vi "washingermmachine.vi"() -> ()   [LabVIEW 2024]
panel:
  out "String 2":string
  out "bytes to read 6":i32
  in  "stop 6":bool
  out "Timer 2":dbl
  out "Water Temp 2":dbl(slide) scale=20.0..60.0
  out "bytes to read 5":i32
  in  "stop 5":bool
  out "Water Level 2":dbl(slide) scale=20.0..60.0
  out "bytes to read 4":i32
  in  "stop 4":bool
  out "Boolean 2":bool
  out "String":string
  out "Timer":dbl
  out "bytes to read 3":i32
  in  "stop 3":bool
  out "Water Temp":dbl(slide) scale=20.0..60.0
  out "bytes to read 2":i32
  in  "stop 2":bool
  in  "stop":bool
  out "bytes to read":i32
  out "Water Level":dbl(slide) scale=20.0..60.0
  out "Boolean":bool
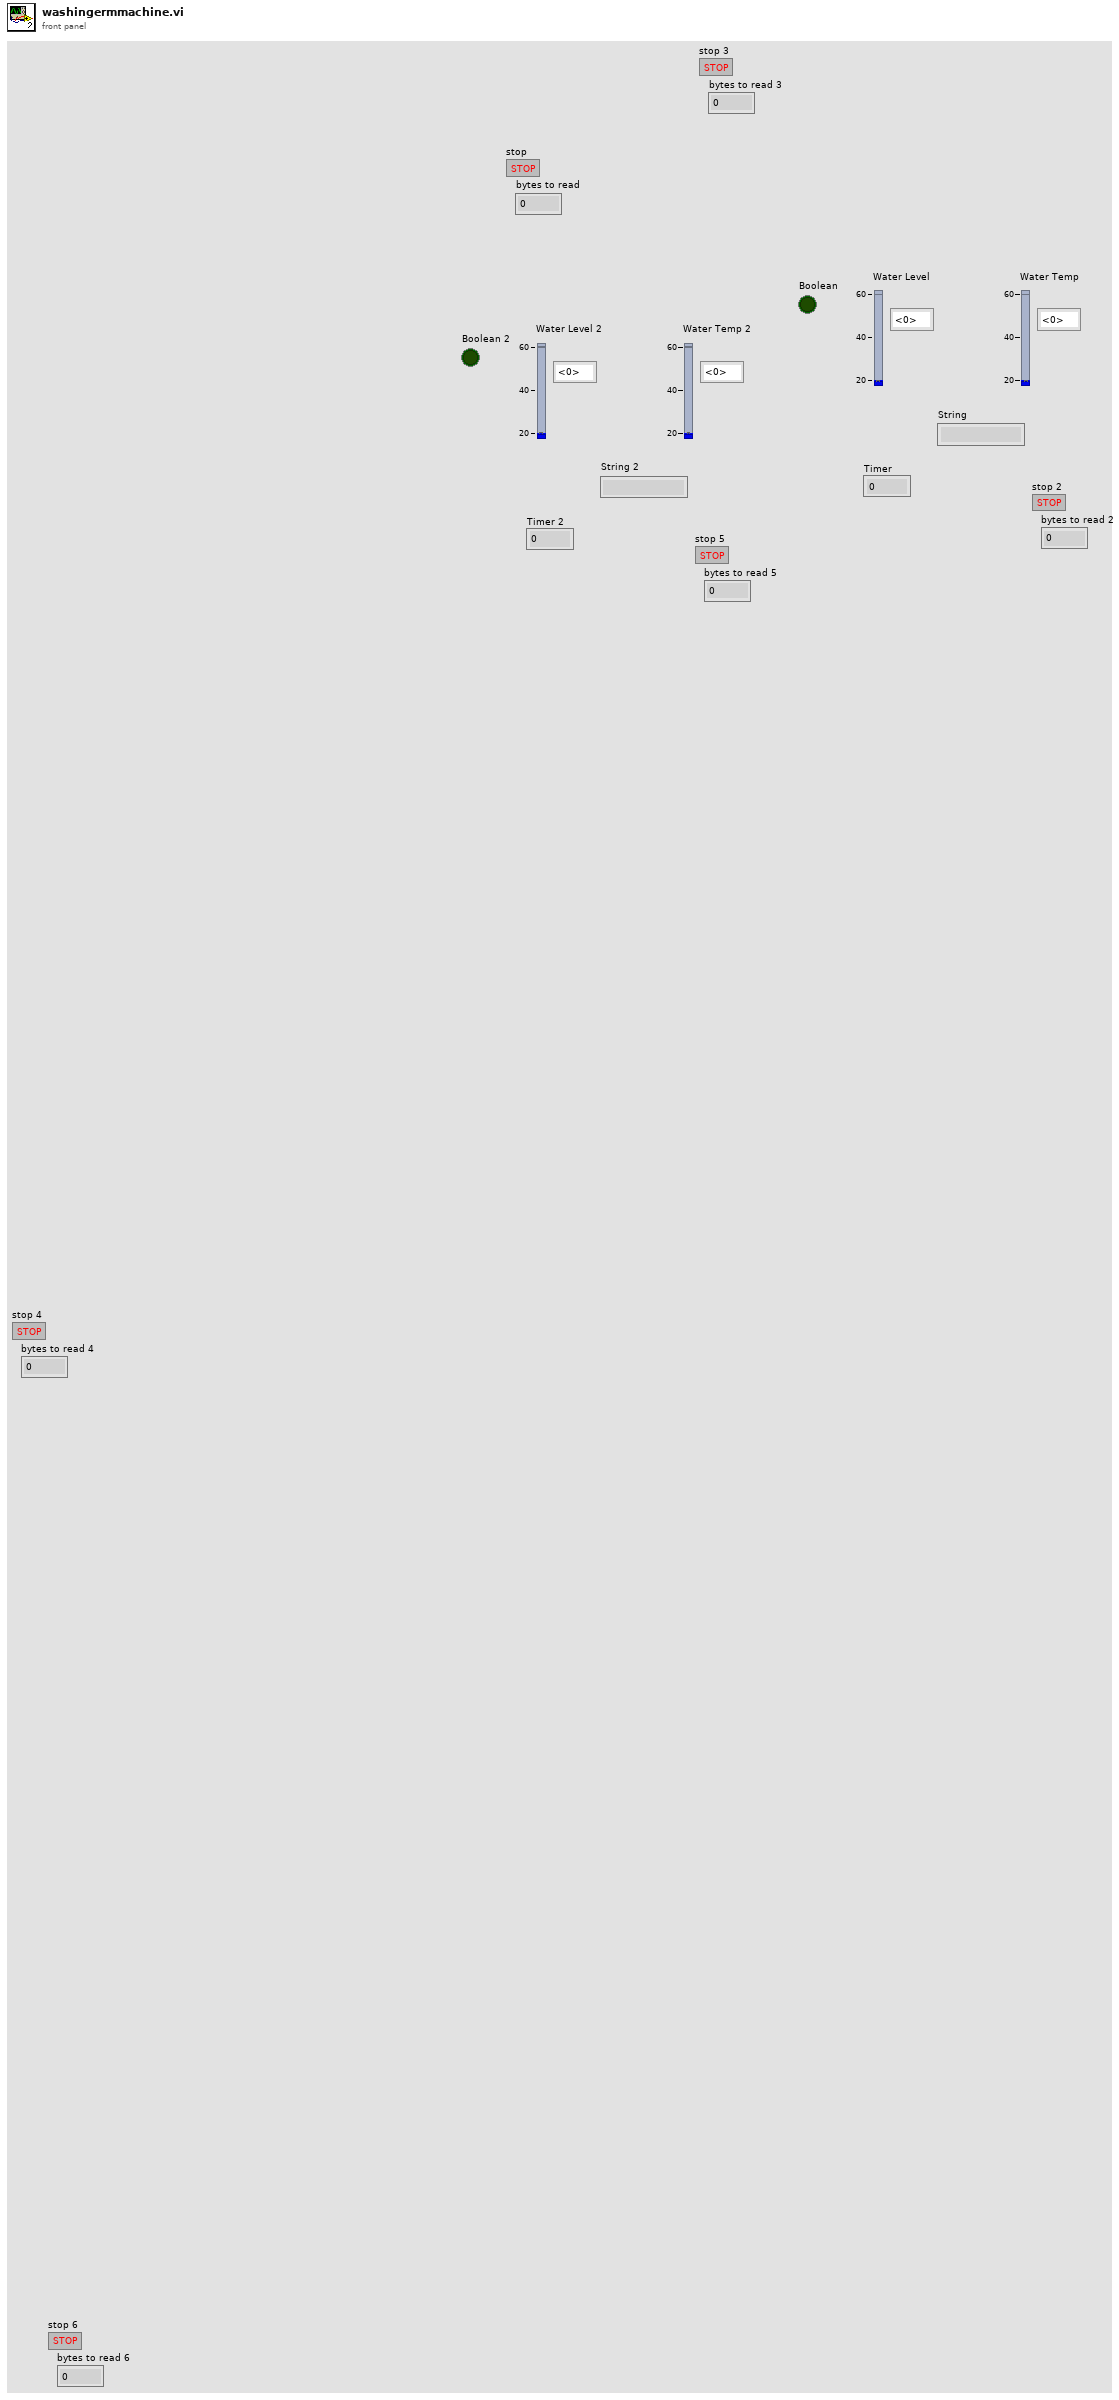
[diagram p1: front panel]
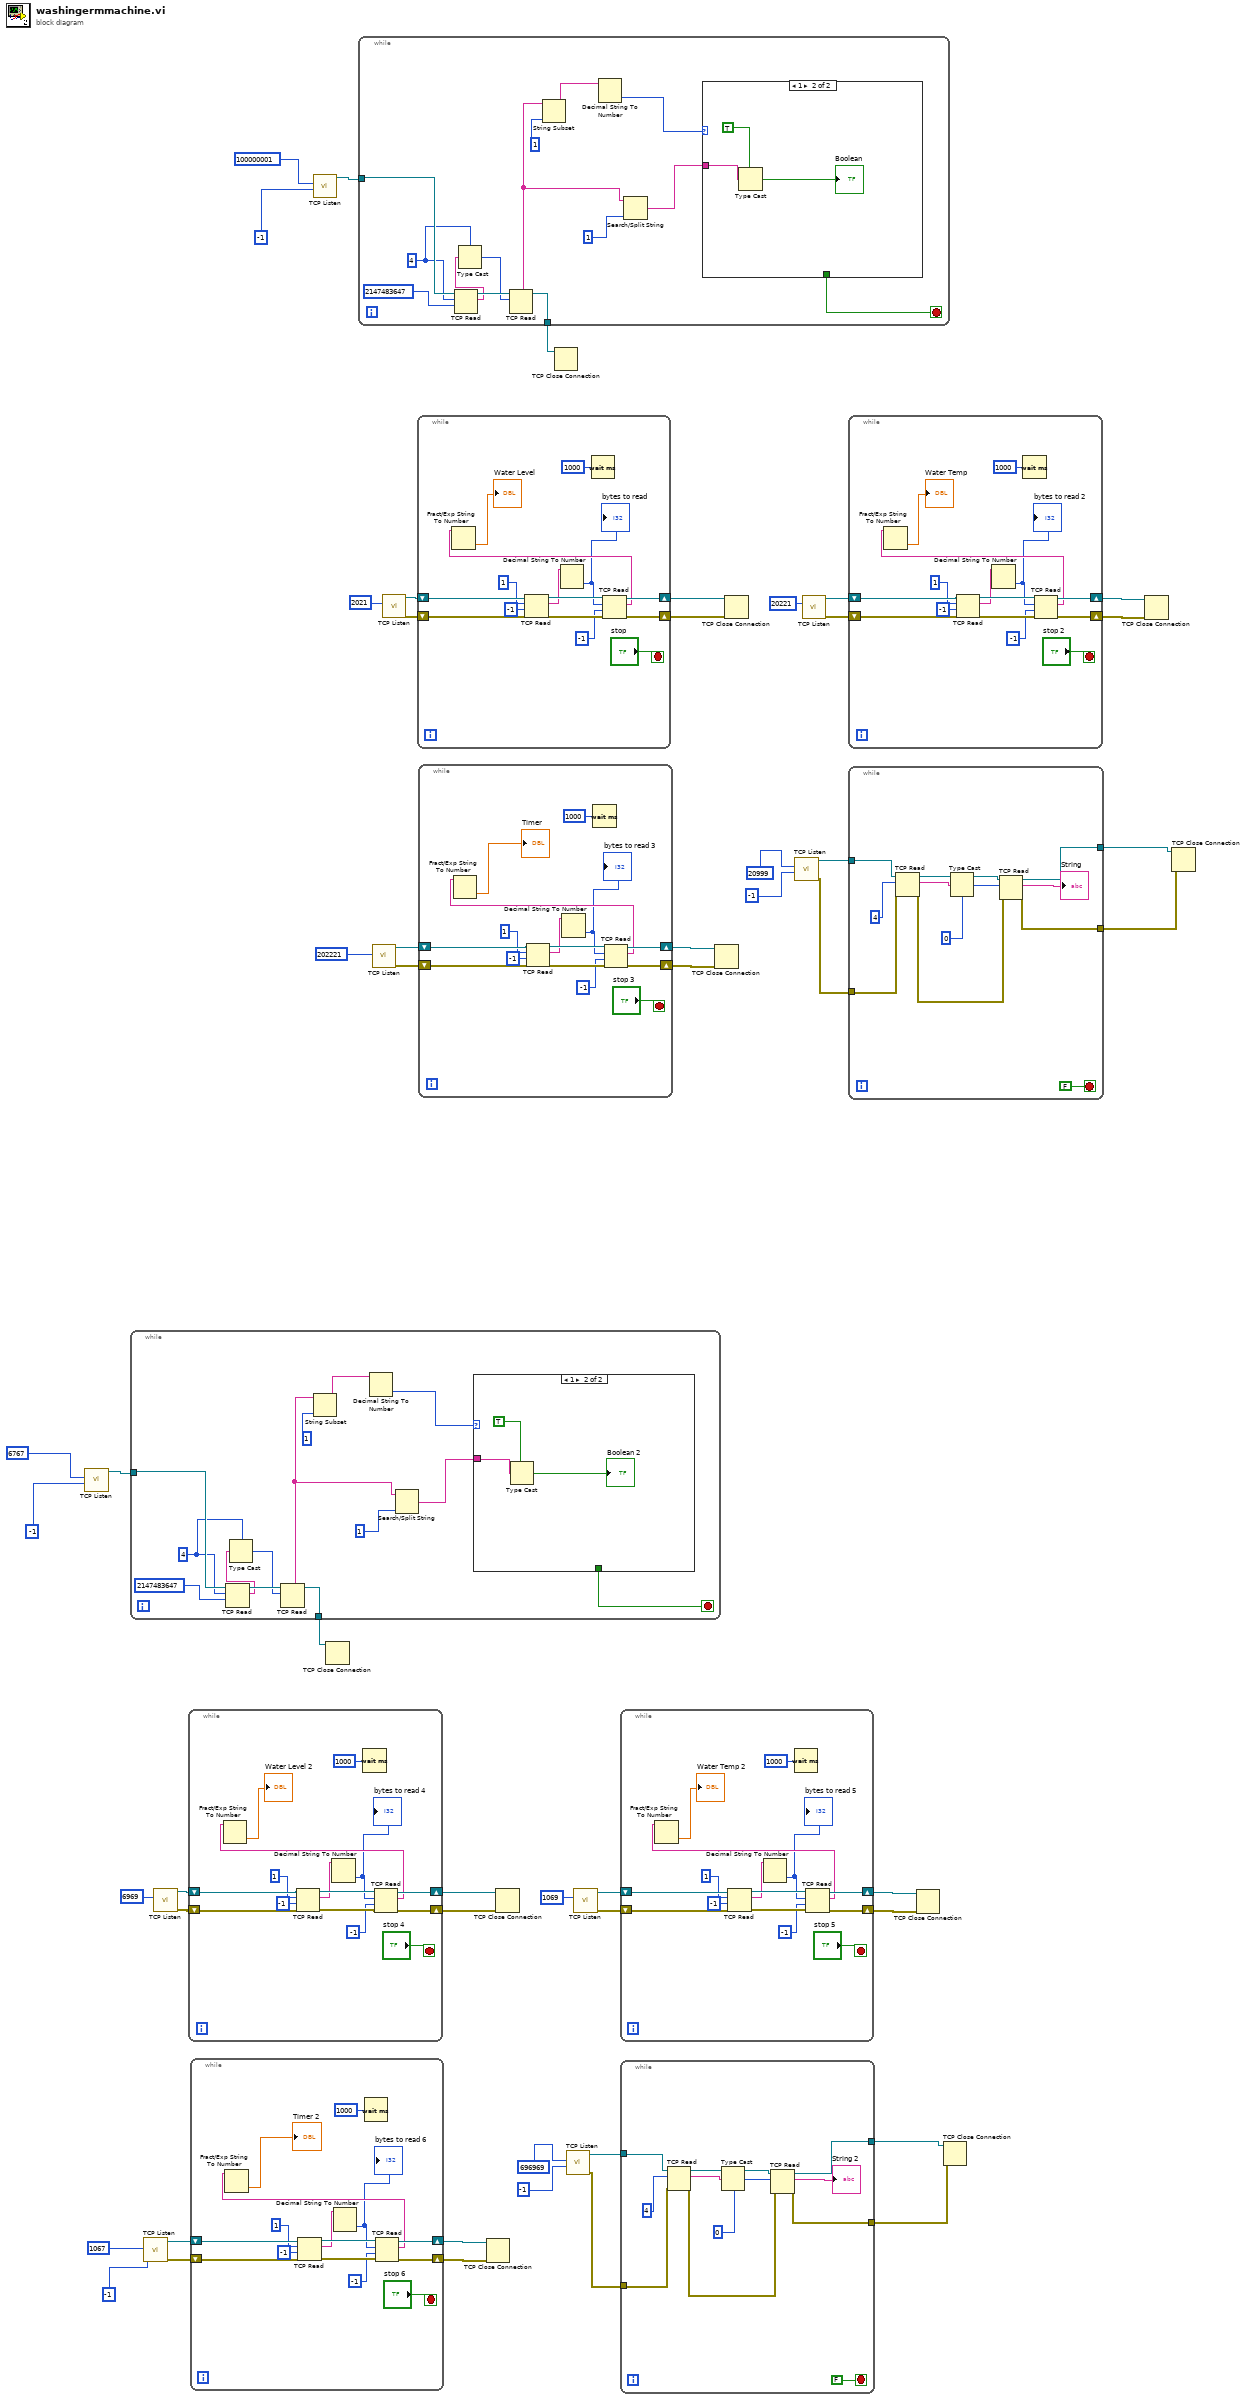
[diagram p0: block diagram]
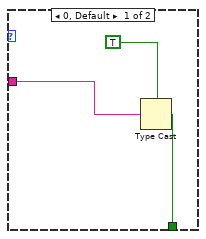
[diagram p2: hidden frame]
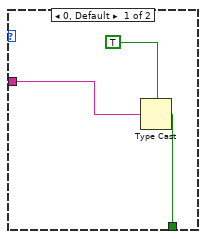
[diagram p3: hidden frame]
diagram:
  n1 = call <vilib>:"TCP Listen.vi"("timeout ms (wait forever: -1)"=-1, "port"=6767) -> ("connection ID"=w24:refnum<k5>)  [unwired: 5 in, 4 out]
  n2 = while {
    tunnel: w24 -> [w65]
    tunnel: [w57] -> w23
    stop <- w58 stop-if-true
    w62 = 4
    n3 = TCP Read(connection ID=w65, bytes to read=w62, 9:2147483647) -> (connection ID out=w64:refnum<k5>, data out=w63:string)  [unwired: 2 in, 1 out]
    n4 = Type Cast(type=w62, x=w63) -> (*(type *) &x=w61:i32)
    n5 = TCP Read(connection ID=w64, bytes to read=w61) -> (connection ID out=w57:refnum<k5>, data out=w54:string)  [unwired: 3 in, 1 out]
    n6 = String Subset(string=w54, length (rest)=1 ("length (rest)")) -> (substring=w55:string)  [unwired: 1 in]
    n7 = Decimal String To Number(string=w55) -> (number=w52:i32)  [unwired: 2 in, 1 out]
    n8 = Search/Split String(string=w54, offset (0)=1) -> (match + rest of string=w59:string)  [unwired: 1 in, 2 out]
    n9 = case shown="1" w52 {
      tunnel: w59 -> [w68 w71]
      tunnel: [w66 _] -> w58
      frame 0, Default {
        n10 = Type Cast(type=TRUE, x=w68) -> (*(type *) &x=w66:bool)
      }
      frame 1 {
        n11 = Type Cast(type=TRUE, x=w71) -> (*(type *) &x=→"Boolean 2":bool)
      }
    }
  }
  n12 = call <vilib>:"TCP Listen.vi"("timeout ms (wait forever: -1)"=-1, "port"=1067) -> ("error out"=w11:errorcluster, "connection ID"=w9:refnum<k5>)  [unwired: 5 in, 3 out]
  n13 = call <vilib>:"TCP Listen.vi"("port"=6969) -> ("error out"=w21:errorcluster, "connection ID"=w19:refnum<k5>)  [unwired: 6 in, 3 out]
  n14 = while {
    shift-right: [w84] -> w20
    shift-left: w19 -> [w86]
    shift-right: [w81] -> w22
    shift-left: w21 -> [w83]
    stop <- "stop 4" stop-if-true
    n15 = TCP Read(connection ID=w86, bytes to read=1, error in (no error)=w83, 9:-1 ("timeout ms (25000)")) -> (connection ID out=w85:refnum<k5>, data out=w78:string, error out=w82:errorcluster)  [unwired: 1 in]
    n16 = Decimal String To Number(string=w78) -> (number=w74:i32)  [unwired: 2 in, 1 out]
    "bytes to read 4" <- w74
    n17 = Wait (ms)(milliseconds to wait=u32 1000) -> ()  [unwired: 1 out]
    n18 = TCP Read(connection ID=w85, bytes to read=w74, error in (no error)=w82, 9:-1 ("timeout ms (25000)")) -> (connection ID out=w84:refnum<k5>, data out=w80:string, error out=w81:errorcluster)  [unwired: 1 in]
    n19 = Fract/Exp String To Number(string=w80) -> (number=→"Water Level 2":dbl)  [unwired: 3 in, 1 out]
  }
  n20 = while {
    shift-right: [w99] -> w10
    shift-left: w9 -> [w101]
    shift-right: [w96] -> w12
    shift-left: w11 -> [w98]
    stop <- "stop 6" stop-if-true
    n21 = TCP Read(connection ID=w101, bytes to read=1, error in (no error)=w98, 9:-1 ("timeout ms (25000)")) -> (connection ID out=w100:refnum<k5>, data out=w94:string, error out=w97:errorcluster)  [unwired: 1 in]
    n22 = Decimal String To Number(string=w94) -> (number=w90:i32)  [unwired: 2 in, 1 out]
    "bytes to read 6" <- w90
    n23 = Wait (ms)(milliseconds to wait=u32 1000) -> ()  [unwired: 1 out]
    n24 = TCP Read(connection ID=w100, bytes to read=w90, error in (no error)=w97, 9:-1 ("timeout ms (25000)")) -> (connection ID out=w99:refnum<k5>, data out=w95:string, error out=w96:errorcluster)  [unwired: 1 in]
    n25 = Fract/Exp String To Number(string=w95) -> (number=→"Timer 2":dbl)  [unwired: 3 in, 1 out]
  }
  n26 = call <vilib>:"TCP Listen.vi"("timeout ms (wait forever: -1)"=-1, "port"=100000001) -> ("connection ID"=w49:refnum<k5>)  [unwired: 5 in, 4 out]
  n27 = TCP Close Connection(connection ID=w23) -> ()  [unwired: 2 in, 2 out]
  n28 = while {
    tunnel: w49 -> [w115]
    tunnel: [w107] -> w48
    stop <- w108 stop-if-true
    w112 = 4
    n29 = TCP Read(connection ID=w115, bytes to read=w112, 9:2147483647) -> (connection ID out=w114:refnum<k5>, data out=w113:string)  [unwired: 2 in, 1 out]
    n30 = Type Cast(type=w112, x=w113) -> (*(type *) &x=w111:i32)
    n31 = TCP Read(connection ID=w114, bytes to read=w111) -> (connection ID out=w107:refnum<k5>, data out=w104:string)  [unwired: 3 in, 1 out]
    n32 = String Subset(string=w104, length (rest)=1 ("length (rest)")) -> (substring=w105:string)  [unwired: 1 in]
    n33 = Decimal String To Number(string=w105) -> (number=w102:i32)  [unwired: 2 in, 1 out]
    n34 = Search/Split String(string=w104, offset (0)=1) -> (match + rest of string=w109:string)  [unwired: 1 in, 2 out]
    n35 = case shown="1" w102 {
      tunnel: w109 -> [w118 w121]
      tunnel: [w116 _] -> w108
      frame 0, Default {
        n36 = Type Cast(type=TRUE, x=w118) -> (*(type *) &x=w116:bool)
      }
      frame 1 {
        n37 = Type Cast(type=TRUE, x=w121) -> (*(type *) &x=→"Boolean":bool)
      }
    }
  }
  n38 = call <vilib>:"TCP Listen.vi"("port"=202221) -> ("error out"=w36:errorcluster, "connection ID"=w34:refnum<k5>)  [unwired: 6 in, 3 out]
  n39 = call <vilib>:"TCP Listen.vi"("port"=2021) -> ("error out"=w46:errorcluster, "connection ID"=w44:refnum<k5>)  [unwired: 6 in, 3 out]
  n40 = while {
    shift-right: [w134] -> w45
    shift-left: w44 -> [w136]
    shift-right: [w131] -> w47
    shift-left: w46 -> [w133]
    stop <- "stop" stop-if-true
    n41 = TCP Read(connection ID=w136, bytes to read=1, error in (no error)=w133, 9:-1 ("timeout ms (25000)")) -> (connection ID out=w135:refnum<k5>, data out=w128:string, error out=w132:errorcluster)  [unwired: 1 in]
    n42 = Decimal String To Number(string=w128) -> (number=w124:i32)  [unwired: 2 in, 1 out]
    "bytes to read" <- w124
    n43 = Wait (ms)(milliseconds to wait=u32 1000) -> ()  [unwired: 1 out]
    n44 = TCP Read(connection ID=w135, bytes to read=w124, error in (no error)=w132, 9:-1 ("timeout ms (25000)")) -> (connection ID out=w134:refnum<k5>, data out=w130:string, error out=w131:errorcluster)  [unwired: 1 in]
    n45 = Fract/Exp String To Number(string=w130) -> (number=→"Water Level":dbl)  [unwired: 3 in, 1 out]
  }
  n46 = while {
    shift-right: [w149] -> w35
    shift-left: w34 -> [w151]
    shift-right: [w146] -> w37
    shift-left: w36 -> [w148]
    stop <- "stop 3" stop-if-true
    n47 = TCP Read(connection ID=w151, bytes to read=1, error in (no error)=w148, 9:-1 ("timeout ms (25000)")) -> (connection ID out=w150:refnum<k5>, data out=w144:string, error out=w147:errorcluster)  [unwired: 1 in]
    n48 = Decimal String To Number(string=w144) -> (number=w140:i32)  [unwired: 2 in, 1 out]
    "bytes to read 3" <- w140
    n49 = Wait (ms)(milliseconds to wait=u32 1000) -> ()  [unwired: 1 out]
    n50 = TCP Read(connection ID=w150, bytes to read=w140, error in (no error)=w147, 9:-1 ("timeout ms (25000)")) -> (connection ID out=w149:refnum<k5>, data out=w145:string, error out=w146:errorcluster)  [unwired: 1 in]
    n51 = Fract/Exp String To Number(string=w145) -> (number=→"Timer":dbl)  [unwired: 3 in, 1 out]
  }
  n52 = TCP Close Connection(connection ID=w10, error in (no error)=w12) -> ()  [unwired: 1 in, 2 out]
  n53 = TCP Close Connection(connection ID=w20, error in (no error)=w22) -> ()  [unwired: 1 in, 2 out]
  n54 = TCP Close Connection(connection ID=w48) -> ()  [unwired: 2 in, 2 out]
  n55 = call <vilib>:"TCP Listen.vi"("timeout ms (wait forever: -1)"=-1, "port"=696969) -> ("error out"=w2:errorcluster, "connection ID"=w7:refnum<k5>)  [unwired: 5 in, 3 out]
  n56 = call <vilib>:"TCP Listen.vi"("port"=1069) -> ("error out"=w16:errorcluster, "connection ID"=w14:refnum<k5>)  [unwired: 6 in, 3 out]
  n57 = while {
    shift-right: [w164] -> w15
    shift-left: w14 -> [w166]
    shift-right: [w161] -> w17
    shift-left: w16 -> [w163]
    stop <- "stop 5" stop-if-true
    n58 = TCP Read(connection ID=w166, bytes to read=1, error in (no error)=w163, 9:-1 ("timeout ms (25000)")) -> (connection ID out=w165:refnum<k5>, data out=w158:string, error out=w162:errorcluster)  [unwired: 1 in]
    n59 = Decimal String To Number(string=w158) -> (number=w154:i32)  [unwired: 2 in, 1 out]
    "bytes to read 5" <- w154
    n60 = Wait (ms)(milliseconds to wait=u32 1000) -> ()  [unwired: 1 out]
    n61 = TCP Read(connection ID=w165, bytes to read=w154, error in (no error)=w162, 9:-1 ("timeout ms (25000)")) -> (connection ID out=w164:refnum<k5>, data out=w160:string, error out=w161:errorcluster)  [unwired: 1 in]
    n62 = Fract/Exp String To Number(string=w160) -> (number=→"Water Temp 2":dbl)  [unwired: 3 in, 1 out]
  }
  n63 = while {
    tunnel: w7 -> [w172]
    tunnel: [w170] -> w4
    tunnel: [w169] -> w3
    tunnel: w2 -> [w167]
    stop <- FALSE stop-if-true
    n64 = TCP Read(connection ID=w172, bytes to read=4, error in (no error)=w167) -> (connection ID out=w171:refnum<k5>, data out=w174:string, error out=w168:errorcluster)  [unwired: 2 in]
    n65 = Type Cast(type=0, x=w174) -> (*(type *) &x=w176:i32)
    n66 = TCP Read(connection ID=w171, bytes to read=w176, error in (no error)=w168) -> (connection ID out=w170:refnum<k5>, data out=→"String 2":string, error out=w169:errorcluster)  [unwired: 2 in]
  }
  n67 = TCP Close Connection(connection ID=w35, error in (no error)=w37) -> ()  [unwired: 1 in, 2 out]
  n68 = TCP Close Connection(connection ID=w45, error in (no error)=w47) -> ()  [unwired: 1 in, 2 out]
  n69 = call <vilib>:"TCP Listen.vi"("timeout ms (wait forever: -1)"=-1, "port"=20999) -> ("error out"=w27:errorcluster, "connection ID"=w32:refnum<k5>)  [unwired: 5 in, 3 out]
  n70 = call <vilib>:"TCP Listen.vi"("port"=20221) -> ("error out"=w41:errorcluster, "connection ID"=w39:refnum<k5>)  [unwired: 6 in, 3 out]
  n71 = while {
    shift-right: [w191] -> w40
    shift-left: w39 -> [w193]
    shift-right: [w188] -> w42
    shift-left: w41 -> [w190]
    stop <- "stop 2" stop-if-true
    n72 = TCP Read(connection ID=w193, bytes to read=1, error in (no error)=w190, 9:-1 ("timeout ms (25000)")) -> (connection ID out=w192:refnum<k5>, data out=w185:string, error out=w189:errorcluster)  [unwired: 1 in]
    n73 = Decimal String To Number(string=w185) -> (number=w181:i32)  [unwired: 2 in, 1 out]
    "bytes to read 2" <- w181
    n74 = Wait (ms)(milliseconds to wait=u32 1000) -> ()  [unwired: 1 out]
    n75 = TCP Read(connection ID=w192, bytes to read=w181, error in (no error)=w189, 9:-1 ("timeout ms (25000)")) -> (connection ID out=w191:refnum<k5>, data out=w187:string, error out=w188:errorcluster)  [unwired: 1 in]
    n76 = Fract/Exp String To Number(string=w187) -> (number=→"Water Temp":dbl)  [unwired: 3 in, 1 out]
  }
  n77 = while {
    tunnel: w32 -> [w199]
    tunnel: [w197] -> w29
    tunnel: [w196] -> w28
    tunnel: w27 -> [w194]
    stop <- FALSE stop-if-true
    n78 = TCP Read(connection ID=w199, bytes to read=4, error in (no error)=w194) -> (connection ID out=w198:refnum<k5>, data out=w201:string, error out=w195:errorcluster)  [unwired: 2 in]
    n79 = Type Cast(type=0, x=w201) -> (*(type *) &x=w203:i32)
    n80 = TCP Read(connection ID=w198, bytes to read=w203, error in (no error)=w195) -> (connection ID out=w197:refnum<k5>, data out=→"String":string, error out=w196:errorcluster)  [unwired: 2 in]
  }
  n81 = TCP Close Connection(connection ID=w15, error in (no error)=w17) -> ()  [unwired: 1 in, 2 out]
  n82 = TCP Close Connection(connection ID=w4, error in (no error)=w3) -> ()  [unwired: 1 in, 2 out]
  n83 = TCP Close Connection(connection ID=w40, error in (no error)=w42) -> ()  [unwired: 1 in, 2 out]
  n84 = TCP Close Connection(connection ID=w29, error in (no error)=w28) -> ()  [unwired: 1 in, 2 out]
